vi "timeout error fg.vi"(0 "Timeout Error?":bool) -> (1 "Time Out Error This Match":bool, 2 "# of Timeouts":u32)   [LabVIEW 2013]
panel:
  # "A Funtctional Global to Store if there has been a Timeout Error"
  # "Very unlike a usual FG"
  # "It writes true if the timeout error control is true,\nbut if it is false it does nothing. This causes a permanent\ntime out error output, which is good, it also displays how\nmany there have been."
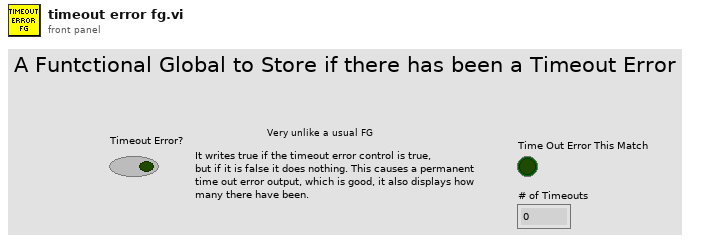
[diagram p1: front panel]
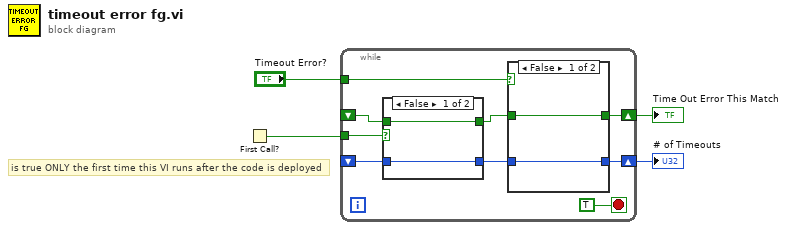
[diagram p0: block diagram]
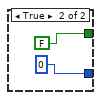
[diagram p2: hidden frame]
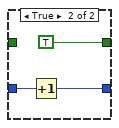
[diagram p3: hidden frame]
diagram:
  # "is true ONLY the first time this VI runs after the code is deployed"
  n1 = First Call?() -> (First Call?: T/F=w1:bool)
  n2 = while {
    shift-right: [w11] -> w3
    shift-left: _ -> [w9]
    tunnel: "Timeout Error?" -> [w12]
    shift-right: [w10] -> w2
    shift-left: _ -> [w7]
    tunnel: w1 -> [w5]
    stop <- TRUE stop-if-true
    n3 = case shown="False" w5 {
      tunnel: w9 -> [w15 _]
      tunnel: [w15 FALSE] -> w8
      tunnel: w7 -> [w14 _]
      tunnel: [w14 u32 0] -> w6
      frame False {
      }
      frame True {
      }
    }
    n4 = case shown="False" w12 {
      tunnel: [w19 TRUE] -> w11
      tunnel: w8 -> [w19 _]
      tunnel: [w18 w20] -> w10
      tunnel: w6 -> [w18 w21]
      frame False {
      }
      frame True {
        n5 = Increment(x=w21) -> (x+1=w20:u32)
      }
    }
  }
  "Time Out Error This Match" <- w3
  "# of Timeouts" <- w2
